vi "LWXPS_PositionerCompensatedFastPCOPulseParametersGet.vi"(0 "XPS Reference IN":refnum<k24>, 7 "Positioner Name":string, 11 "LabVIEW error IN":errorcluster) -> (3 "XPS Reference OUT":refnum<k24>, 4 "Returned error code":i32, 6 "Pulse width":dbl, 8 "Pulse polarity":i32, 10 "Pulse toggle":bool, 14 "LabVIEW error OUT":errorcluster, 15 "XPS Error String":string)   [LabVIEW 2014]
uses:
  D:/XPSQ8_LabView_Library/Development/Source/Dll/Newport.XPS.CommandInterface.dll
  Dll/Newport.XPS.CommandInterface.dll
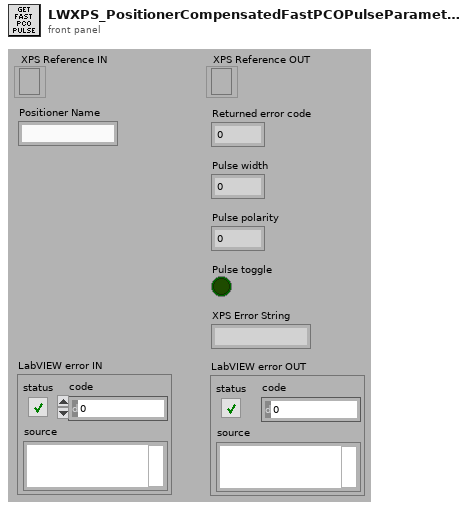
[diagram p1: front panel]
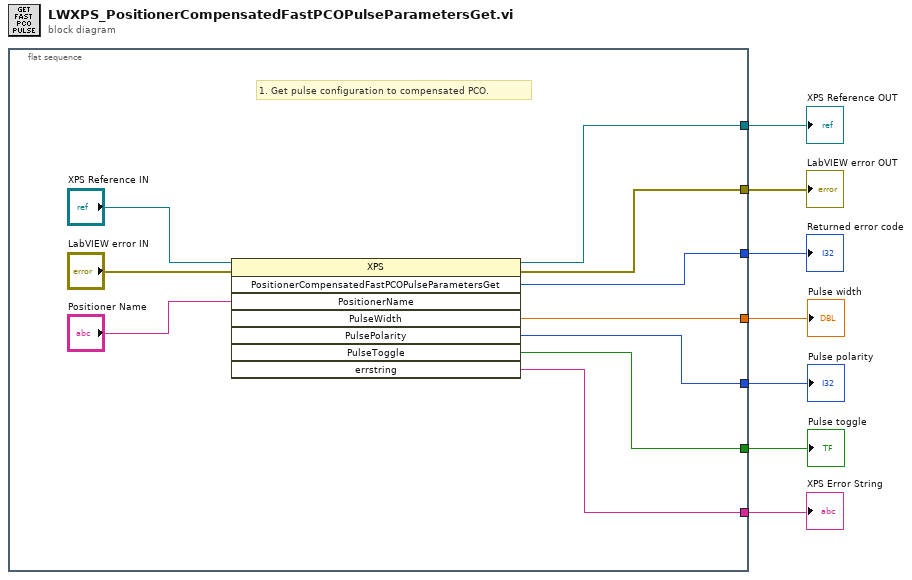
[diagram p0: block diagram]
diagram:
  n1 = flat-sequence {
    tunnel: [w15] -> w7
    tunnel: [w12] -> w6
    tunnel: [w16] -> w5
    tunnel: [w10] -> w3
    tunnel: [w11] -> w2
    tunnel: [w9] -> w1
    tunnel: [w8] -> w4
    frame #0 {
      # "1. Get pulse configuration to compensated PCO."
      n2 = invoke class="XPS" method="PositionerCompensatedFastPCOPulseParametersGet"(reference="XPS Reference IN", error in="LabVIEW error IN", "PositionerName"="Positioner Name") -> (reference out=w15:refnum<k24>, error out=w12:errorcluster, "PositionerCompensatedFastPCOPulseParametersGet"=w16:i32, "PulseWidth"=w10:dbl, "PulsePolarity"=w11:i32, "PulseToggle"=w9:bool, "errstring"=w8:string)  [unwired: 5 in, 1 out]
    }
  }
  "XPS Error String" <- w4
  "XPS Reference OUT" <- w7
  "LabVIEW error OUT" <- w6
  "Returned error code" <- w5
  "Pulse width" <- w3
  "Pulse polarity" <- w2
  "Pulse toggle" <- w1
